vi "Initialize-motors.vi"(8 "error in (no error)":errorcluster, 11 "Object ref in":T1) -> (0 "error out":errorcluster, 3 "Object ref out":T1)   [LabVIEW 2013]
uses:
  PD-PowderDeposition/Sources/Assembly/Motor-assembly.lvclass
  BC-Main.lvclass
  Object-reference.ctl
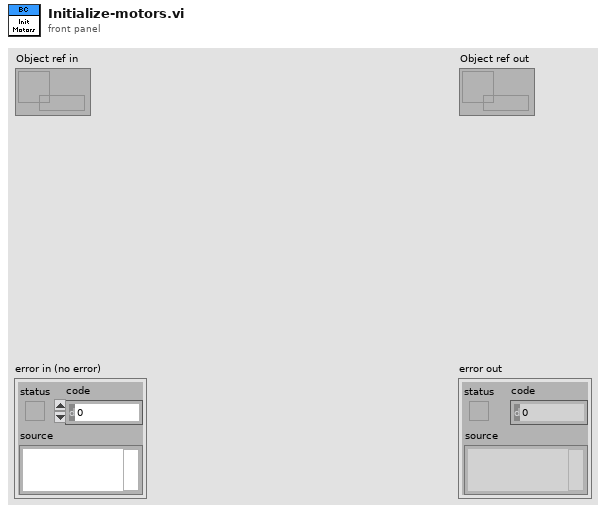
[diagram p1: front panel]
types:
  T1 = typedef "BeamControl.lvlib/BC-Main.lvclass/Object-reference.ctl" = refnum<data-value>
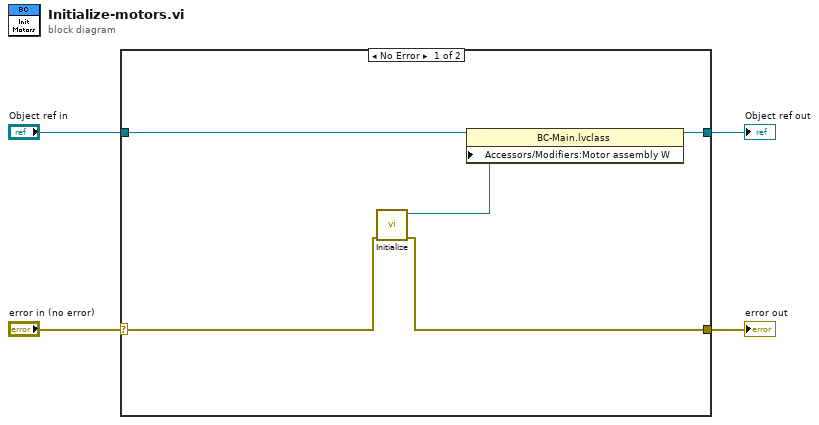
[diagram p0: block diagram]
diagram:
  n1 = case shown="No Error" "error in (no error)" {
    selector: "error in (no error)" -> [w6 w11]
    tunnel: [w5 w11] -> w3
    tunnel: [w8 w10] -> w1
    tunnel: "Object ref in" -> [w9 w10]
    frame No Error {
      n2 = call "Initialize.vi"("error in (no error)"=w6) -> ("error out"=w5:errorcluster, "Available motors out"=w7:refnum<class "Motor-assembly.lvclass">)  [unwired: 9 in]
      n3 = property class="BC-Main.lvclass"(reference=w9, "Accessors/Modifiers:Motor assembly W"=w7) -> (reference out=w8:T1)  [unwired: 1 in, 1 out]
    }
    frame Error {
    }
  }
  "error out" <- w3
  "Object ref out" <- w1
